vi "Get ChanGrp Members.vi"(8 "error in":errorcluster, 9 "Channel Groups":T1, 11 "Chassis Cfg":refnum<class "ChassisCfg.lvclass">) -> (0 "error out":errorcluster, 2 "Group Members":string[][](array[string]), 3 "Chassis Cfg":refnum<class "ChassisCfg.lvclass">)   [LabVIEW 2018, in "Configuration Grandmaster.lvlib" / "ChassisCfg.lvclass"]
uses:
  ChassisCfg.lvclass
  Common/Controls/Selected Group.ctl
  Common/Controls/TE_Designator.ctl
  ChassisCfg.lvclass/ChassisCfg.ctl
  Class Timing Group/TimingGrp.lvclass
  Class Chan Group/ChanGrp.lvclass
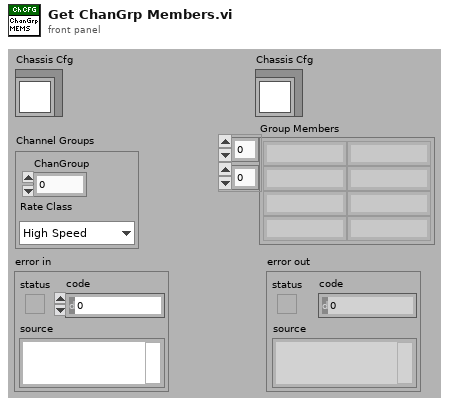
[diagram p1: front panel]
types:
  T1 = typedef "Selected Group.ctl" = cluster{"ChanGroup":i32, "Rate Class":T2}
  T2 = typedef "TE_Designator.ctl" = enum16{"High Speed", "Low Speed"}
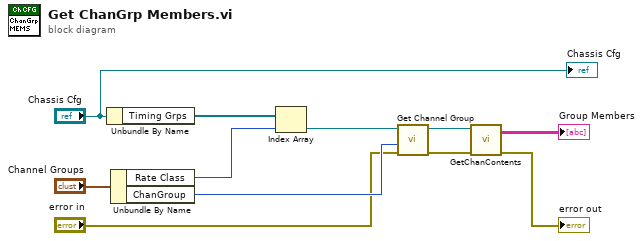
[diagram p0: block diagram]
diagram:
  n1 = Unbundle By Name("Chassis Cfg") -> ("Timing Grps"=w4:refnum<class "TimingGrp.lvclass">[])
  n2 = Unbundle By Name("Channel Groups") -> ("Rate Class"=w3:T2, "ChanGroup"=w10:i32)
  n3 = Index Array(array=w4, index=w3) -> (element=w2:refnum<class "TimingGrp.lvclass">)
  n4 = call "Get Channel Group.vi"("error in (no error)"="error in", "ChanGroup"=w10, "TimingGrp in"=w2) -> ("error out"=w7:errorcluster, "Chan Gropu"=w8:refnum<class "ChanGrp.lvclass">)  [unwired: 7 in]
  n5 = call "GetChanContents.vi"("error in"=w7, "ChanGrp.lvclass"=w8) -> ("error out"=→"error out":errorcluster, "Chan Aliases"=→"Group Members":string[][])  [unwired: 3 in, 5 out]
  "Chassis Cfg" <- "Chassis Cfg"
